vi "Periodic Tasks.vi"   [LabVIEW 2011]
doc: "This VI runs in parallel to other tasks. It can contain as many user-defined periodic loops as you need. These can carry out PID or other sorts of timed response."
uses:
  <vilib>/Rock Robotics/SystemInterfaces/Utilities/FPGA_UtilitiesLED State.ctl
  <vilib>/Rock Robotics/SystemInterfaces/Utilities/FPGA_UtilitiesLED Source.ctl
  <vilib>/Rock Robotics/WPI/Relay/WPI_RelayValue.ctl
  <vilib>/Rock Robotics/WPI/Solenoid/WPI_SolenoidValue.ctl
  System Set Points and States.vi
  <vilib>/Rock Robotics/WPI/Solenoid/WPI_SolenoidSetEnum.vi
  <vilib>/Rock Robotics/WPI/Compressor/WPI_CompressorGetSetRefNum.vi
  Robot Global Data.vi
types:
  T1 = typedef "WPI_RelayValue.ctl" = enum16{"Off", "On", "Forward", "Reverse"}
  T2 = typedef "WPI_SolenoidValue.ctl" = enum16{"Off", "On", "Forward", "Reverse"}
  T3 = typedef "WPI_DigitalInputDevRef.ctl" = cluster{"DevStatus":errorcluster, "DIO Channel":T4, "Digital Module":T5}
  T4 = typedef "FPGA_DIOChannel.ctl" = enum8{"DIO 1", "DIO 2", "DIO 3", "DIO 4", "DIO 5", "DIO 6", "DIO 7", "DIO 8", "DIO 9", "DIO 10", "DIO 11", "DIO 12", "DIO 13", "DIO 14", "Invalid"}
  T5 = typedef "FPGA_TypedefDigitalModule.ctl" = enum16{"Digital Module 1", "Digital Module 2"}
  T6 = typedef "WPI_RelayDevRef.ctl" = cluster{"DevStatus":errorcluster, "Relay Channel":T7, "Digital Module":T5, "Relay Direction":T8}
  T7 = typedef "FPGA_DIORelayChannel.ctl" = enum8{"Relay 1", "Relay 2", "Relay 3", "Relay 4", "Relay 5", "Relay 6", "Relay 7", "Relay 8", "Invalid"}
  T8 = typedef "WPI_RelayDirection.ctl" = enum16{"Both directions", "Forward only", "Reverse only"}
  T9 = typedef "WPI_SolenoidDevRef.ctl" = cluster{"DevStatus":errorcluster, "Solenoid Module":T10, "Forward Solenoid Channel":T11, "Reverse Solenoid Channel":T11}
  T10 = typedef "FPGA_TypedefSolenoidModule.ctl" = enum16{"Solenoid Module 1", "Solenoid Module 2"}
  T11 = typedef "WPI_SolenoidChannel.ctl" = enum8{"Solenoid 1", "Solenoid 2", "Solenoid 3", "Solenoid 4", "Solenoid 5", "Solenoid 6", "Solenoid 7", "Solenoid 8", "Invalid"}
  T12 = typedef "WPI_MotorControlDeviceRef.ctl" = cluster{"DeviceStatus":errorcluster, "Type":enum16{"PWM", "CAN"}, "PWM":cluster{"Digital Module":T5, "PWM Channel":T13, "DeadBand":T14}, "CAN":cluster{"Device Number":u8, "Control Mode":T15, "Semaphore":T16, "Max Vout":dbl}, "Invert":bool, "TransformRef":T17, "InvTransformRef":T17}
  T13 = typedef "FPGA_DIOPWMChannel.ctl" = enum8{"PWM 1", "PWM 2", "PWM 3", "PWM 4", "PWM 5", "PWM 6", "PWM 7", "PWM 8", "PWM 9", "PWM 10", "Invalid"}
  T14 = typedef "WPI_PWMDeadband.ctl" = cluster{"Name":string, "maxPositivePwm":i32, "minPositivePwm":i32, "centerPwm":i32, "maxNegativePwm":i32, "minNegativePwm":i32, "angularRange":u16}
  T15 = typedef "WPI_CANJaguar_ControlMode.ctl" = enum8{"Percent VBus", "Current", "Speed", "Position", "Voltage"}
  T16 = typedef "Semaphore RefNum" = refnum<k1>
  T17 = typedef "WPI_PWMTransform_ConPane.ctl" = refnum<vi>
  T18 = typedef "WPI_CompressorDevRef.ctl" = cluster{"DevStatus":errorcluster, "DigitalInputDevRef":T3, "RelayDevRef":T6}
  T19 = typedef "FPGA_UtilitiesLED State.ctl" = enum16{"Off", "On", "Toggle"}
  T20 = typedef "FPGA_UtilitiesLED Source.ctl" = enum16{"User LED", "FPGA LED"}
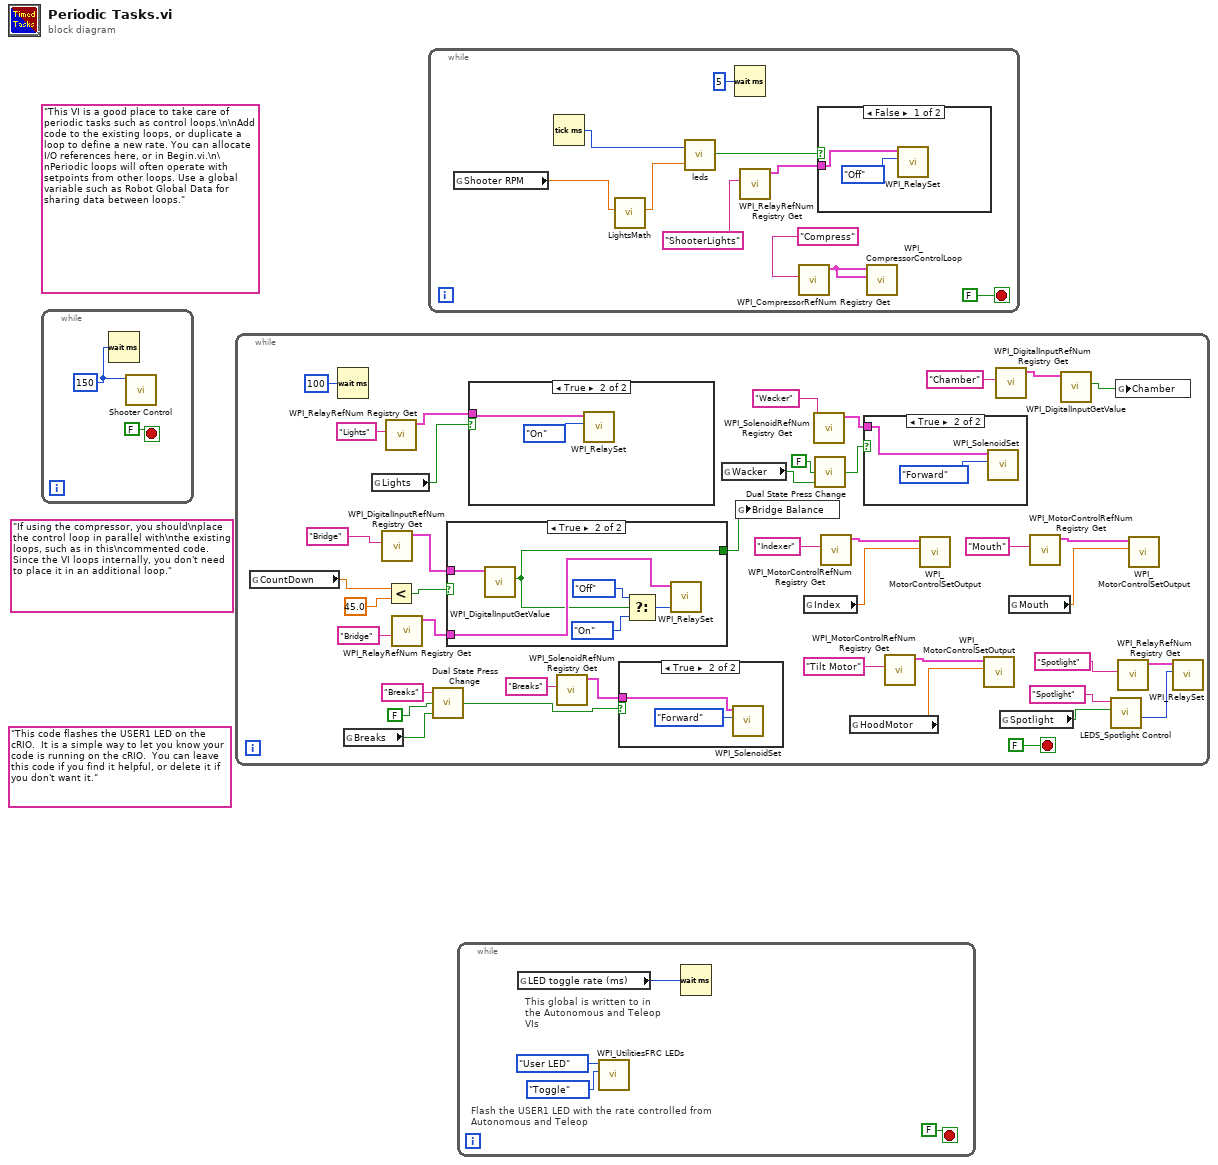
[diagram p0: block diagram]
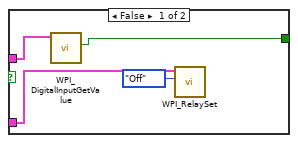
[diagram p2: hidden frame]
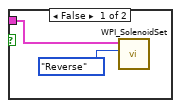
[diagram p3: hidden frame]
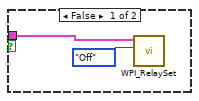
[diagram p4: hidden frame]
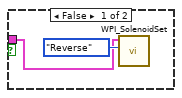
[diagram p5: hidden frame]
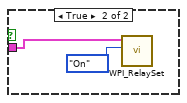
[diagram p6: hidden frame]
diagram:
  (unwired) "If using the compressor, you should\nplace the control loop in parallel with\nthe existing loops, such as in this\ncommented code. Since the VI loops internally, you don't need to place it in an additional loop."
  (unwired) "This code flashes the USER1 LED on the cRIO.  It is a simple way to let you know your code is running on the cRIO.  You can leave this code if you find it helpful, or delete it if you don't want it."
  (unwired) "This VI is a good place to take care of periodic tasks such as control loops.\n\nAdd code to the existing loops, or duplicate a loop to define a new rate. You can allocate I/O references here, or in Begin.vi.\n\nPeriodic loops will often operate with setpoints from other loops. Use a global variable such as Robot Global Data for sharing data between loops."
  n1 = while {
    stop <- FALSE stop-if-true
    w1 = u32 150 ("milliseconds to wait")
    n2 = Wait (ms)(milliseconds to wait=w1) -> ()  [unwired: 1 out]
    n3 = call "Shooter Control.vi"("Time Delay Milli"=w1) -> ()  [unwired: 11 in]
  }
  n4 = while {
    stop <- FALSE stop-if-true
    n5 = global read "System Set Points and States.vi" "CountDown"() -> (w22:dbl)
    n6 = Wait (ms)(milliseconds to wait=u32 100) -> ()  [unwired: 1 out]
    n7 = global read "System Set Points and States.vi" "Breaks"() -> (w9:bool)
    n8 = global read "System Set Points and States.vi" "Lights"() -> (w27:bool)
    n9 = call <vilib>:"WPI_DigitalInputRefNum Registry Get.vi"("refnum name"="Bridge") -> ("DigitalInputDevRef"=w15:T3)  [unwired: 9 in, 1 out]
    n10 = call <vilib>:"WPI_RelayRefNum Registry Get.vi"("refnum name"="Lights") -> ("RelayDevRef"=w25:T6)  [unwired: 9 in, 1 out]
    n11 = Less?(x=w22, y=45.0) -> (x < y?=w17:bool)
    n12 = call <vilib>:"WPI_RelayRefNum Registry Get.vi"("refnum name"="Bridge") -> ("RelayDevRef"=w19:T6)  [unwired: 9 in, 1 out]
    n13 = call "Dual State Press Change.vi"("Enable/Disable"=w9, "Initial"=FALSE, "Value Name"="Breaks") -> ("Enabled"=w8:bool)
    n14 = case shown="True" w17 {
      tunnel: w15 -> [w45 w53]
      tunnel: w19 -> [w47 w49]
      tunnel: [w44 w48] -> w21
      frame False {
        n15 = call <vilib>:"WPI_DigitalInputGetValue.vi"("DigitalInputDevRef"=w45) -> ("Value"=w44:bool)  [unwired: 8 in, 2 out]
        n16 = call <vilib>:"WPI_RelaySet.vi"("RelayValue"=WPI_RelayValue."Off", "RelayDevRef"=w47) -> ()  [unwired: 8 in, 2 out]
      }
      frame True {
        n17 = call <vilib>:"WPI_DigitalInputGetValue.vi"("DigitalInputDevRef"=w53) -> ("Value"=w48:bool)  [unwired: 8 in, 2 out]
        n18 = Select(t=WPI_RelayValue."Off" ("Relay State"), s=w48, f=WPI_RelayValue."On" ("Relay State")) -> (s? t:f=w52:T1)
        n19 = call <vilib>:"WPI_RelaySet.vi"("RelayValue"=w52, "RelayDevRef"=w49) -> ()  [unwired: 8 in, 2 out]
      }
    }
    n20 = case shown="True" w27 {
      tunnel: w25 -> [w59 w61]
      frame False {
        n21 = call <vilib>:"WPI_RelaySet.vi"("RelayValue"=WPI_RelayValue."Off", "RelayDevRef"=w59) -> ()  [unwired: 8 in, 2 out]
      }
      frame True {
        n22 = call <vilib>:"WPI_RelaySet.vi"("RelayValue"=WPI_RelayValue."On", "RelayDevRef"=w61) -> ()  [unwired: 8 in, 2 out]
      }
    }
    n23 = call <vilib>:"WPI_SolenoidRefNum Registry Get.vi"("refnum name"="Breaks") -> ("SolenoidDevRef"=w33:T9)  [unwired: 9 in, 1 out]
    n24 = case shown="True" w8 {
      tunnel: w33 -> [w62 w64]
      frame False {
        n25 = call-poly <vilib>:"WPI_SolenoidSet.vi"("Value"=WPI_SolenoidValue."Reverse", "SolenoidDevRef"=w62) -> ()  [unwired: 8 in, 2 out]
      }
      frame True {
        n26 = call-poly <vilib>:"WPI_SolenoidSet.vi"("Value"=WPI_SolenoidValue."Forward", "SolenoidDevRef"=w64) -> ()  [unwired: 8 in, 2 out]
      }
    }
    n27 = global read "System Set Points and States.vi" "Wacker"() -> (w12:bool)
    n28 = global write "System Set Points and States.vi" "Bridge Balance"(w21) -> ()
    n29 = global read "System Set Points and States.vi" "Index"() -> (w41:dbl)
    n30 = call <vilib>:"WPI_SolenoidRefNum Registry Get.vi"("refnum name"="Wacker") -> ("SolenoidDevRef"=w24:T9)  [unwired: 9 in, 1 out]
    n31 = call "Dual State Press Change.vi"("Enable/Disable"=w12, "Initial"=FALSE) -> ("Enabled"=w10:bool)  [unwired: 1 in]
    n32 = call <vilib>:"WPI_MotorControlRefNum Registry Get.vi"("refnum name"="Indexer") -> ("MotorControlDevRef"=w42:T12)  [unwired: 9 in, 1 out]
    n33 = global read "System Set Points and States.vi" "HoodMotor"() -> (w37:dbl)
    n34 = case shown="True" w10 {
      tunnel: w24 -> [w55 w56]
      frame False {
        n35 = call-poly <vilib>:"WPI_SolenoidSet.vi"("Value"=WPI_SolenoidValue."Reverse", "SolenoidDevRef"=w55) -> ()  [unwired: 8 in, 2 out]
      }
      frame True {
        n36 = call-poly <vilib>:"WPI_SolenoidSet.vi"("Value"=WPI_SolenoidValue."Forward", "SolenoidDevRef"=w56) -> ()  [unwired: 8 in, 2 out]
      }
    }
    n37 = call <vilib>:"WPI_MotorControlRefNum Registry Get.vi"("refnum name"="Tilt Motor") -> ("MotorControlDevRef"=w36:T12)  [unwired: 9 in, 1 out]
    n38 = call <vilib>:"WPI_MotorControlSetOutput.vi"("Output"=w41, "MotorControlDevRef"=w42) -> ()  [unwired: 8 in, 2 out]
    n39 = call <vilib>:"WPI_MotorControlSetOutput.vi"("Output"=w37, "MotorControlDevRef"=w36) -> ()  [unwired: 8 in, 2 out]
    n40 = call <vilib>:"WPI_DigitalInputRefNum Registry Get.vi"("refnum name"="Chamber") -> ("DigitalInputDevRef"=w4:T3)  [unwired: 9 in, 1 out]
    n41 = global read "System Set Points and States.vi" "Spotlight"() -> (w32:bool)
    n42 = global read "System Set Points and States.vi" "Mouth"() -> (w38:dbl)
    n43 = call <vilib>:"WPI_MotorControlRefNum Registry Get.vi"("refnum name"="Mouth") -> ("MotorControlDevRef"=w39:T12)  [unwired: 9 in, 1 out]
    n44 = call <vilib>:"WPI_DigitalInputGetValue.vi"("DigitalInputDevRef"=w4) -> ("Value"=w3:bool)  [unwired: 8 in, 2 out]
    n45 = call "LEDS_Spotlight Control.vi"("Name"="Spotlight", "Button"=w32) -> ("Relay State"=w30:T1)  [unwired: 8 in]
    n46 = global write "System Set Points and States.vi" "Chamber"(w3) -> ()
    n47 = call <vilib>:"WPI_RelayRefNum Registry Get.vi"("refnum name"="Spotlight") -> ("RelayDevRef"=w28:T6)  [unwired: 9 in, 1 out]
    n48 = call <vilib>:"WPI_MotorControlSetOutput.vi"("Output"=w38, "MotorControlDevRef"=w39) -> ()  [unwired: 8 in, 2 out]
    n49 = call <vilib>:"WPI_RelaySet.vi"("RelayValue"=w30, "RelayDevRef"=w28) -> ()  [unwired: 8 in, 2 out]
  }
  n50 = while {
    stop <- FALSE stop-if-true
    n51 = global read "System Set Points and States.vi" "Shooter RPM"() -> (w73:dbl)
    n52 = Tick Count (ms)() -> (millisecond timer value=w75:u32)
    n53 = call "LightsMath.vi"("Shooter RPM"=w73) -> ("Light Timing"=w72:dbl)  [unwired: 10 in]
    n54 = call "leds.vi"("range (centisec)"=w72, "input"=w75) -> ("Output"=w70:bool)
    n55 = Wait (ms)(milliseconds to wait=u32 5) -> ()  [unwired: 1 out]
    n56 = call <vilib>:"WPI_RelayRefNum Registry Get.vi"("refnum name"="ShooterLights") -> ("RelayDevRef"=w71:T6)  [unwired: 9 in, 1 out]
    n57 = call <vilib>:"WPI_CompressorRefNum Registry Get.vi"("refnum name"="Compress") -> ("CompressorDevRef"=w66:T18)  [unwired: 9 in, 1 out]
    n58 = case shown="False" w70 {
      tunnel: w71 -> [w76 w78]
      frame False {
        n59 = call <vilib>:"WPI_RelaySet.vi"("RelayValue"=WPI_RelayValue."Off", "RelayDevRef"=w76) -> ()  [unwired: 8 in, 2 out]
      }
      frame True {
        n60 = call <vilib>:"WPI_RelaySet.vi"("RelayValue"=WPI_RelayValue."On", "RelayDevRef"=w78) -> ()  [unwired: 8 in, 2 out]
      }
    }
    n61 = call <vilib>:"WPI_CompressorControlLoop.vi"("CompressorDevRef 2"=w66, "CompressorDevRef"=w66) -> ()  [unwired: 10 in]
  }
  n62 = while {
    stop <- FALSE stop-if-true
    # "This global is written to in the Autonomous and Teleop VIs"
    # "Flash the USER1 LED with the rate controlled from Autonomous and Teleop"
    n63 = global read "Robot Global Data.vi" "LED toggle rate (ms)"() -> (w80:u32)
    n64 = call <vilib>:"WPI_UtilitiesFRC LEDs.vi"("State"=FPGA_UtilitiesLED_State."Toggle", "LED Type"=FPGA_UtilitiesLED_Source."User LED") -> ()  [unwired: 1 in, 9 out]
    n65 = Wait (ms)(milliseconds to wait=w80) -> ()  [unwired: 1 out]
  }
